vi "Release-all-files.vi"(8 "error in (no error)":errorcluster, 11 "Data ref. in":refnum<data-value>) -> (0 "error out":errorcluster, 3 "Data ref.":refnum<data-value>, 5 "Success?":bool)   [LabVIEW 2013, in "CameraVision.lvlib" / "CV-Main.lvclass"]
uses:
  CV-Main.lvclass
  CV-Main.lvclass/CV-Main.ctl
  Read Storage params.vi
  Storage/CV-Storage.lvclass
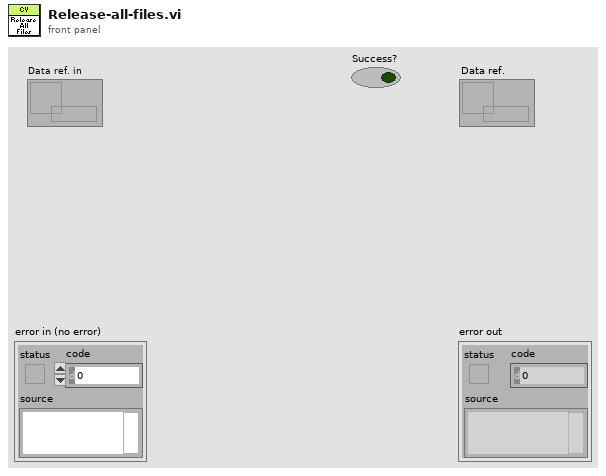
[diagram p1: front panel]
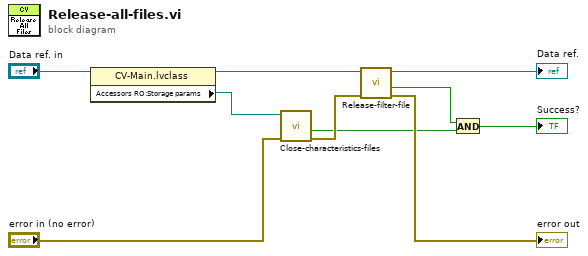
[diagram p0: block diagram]
diagram:
  n1 = property class="CV-Main.lvclass"(reference="Data ref. in") -> (reference out=w5:refnum<data-value>, "Accessors RO:Storage params"=w3:refnum<data-value>)  [unwired: 1 in, 1 out]
  n2 = call "Close-characteristics-files.vi"("error in"="error in (no error)", "Storage params. ref. in"=w3) -> ("error IO"=w4:errorcluster, "Succes?"=w2:bool)  [unwired: 7 in, 1 out]
  n3 = call "Release-filter-file.vi"("error in"=w4, "Data ref. in"=w5) -> ("error IO"=→"error out":errorcluster, "Succes?"=w1:bool, "Data ref."=→"Data ref.":refnum<data-value>)  [unwired: 7 in]
  n4 = And(x=w1, y=w2) -> (x .and. y?=→"Success?":bool)
